vi "NIDAQControl.vi"() -> ()   [LabVIEW 2015]
uses:
  <vilib>/Analysis/NI_AALBase.lvlib
  NIDAQGlobals.vi
  <vilib>/Analysis/baseanly.llb/Mean (DBL).vi
  <vilib>/DAQmx/write.llb/DAQmx Write (Analog 1D Wfm NChan NSamp).vi
panel:
  in  "error out":errorcluster
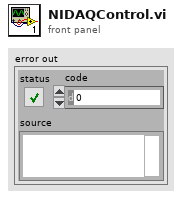
[diagram p1: front panel]
types:
  T1 = typedef "Rendezvous RefNum" = refnum<k1>
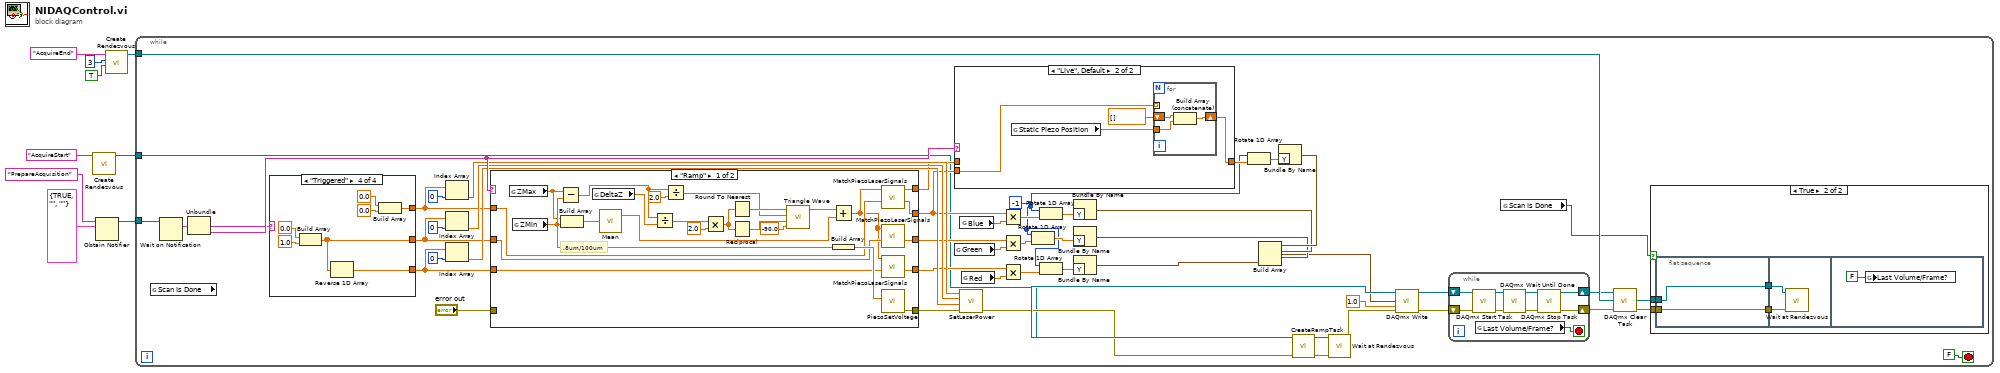
[diagram p0: block diagram]
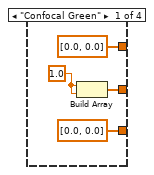
[diagram p4: hidden frame]
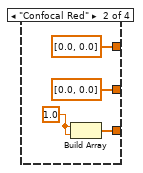
[diagram p5: hidden frame]
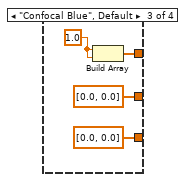
[diagram p6: hidden frame]
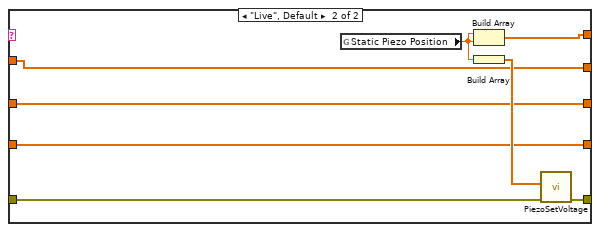
[diagram p7: hidden frame]
diagram:
  n1 = call <vilib>:"Create Rendezvous.vi"("name (unnamed)"="AcquireStart") -> ("rendezvous"=w5:T1)  [unwired: 4 in, 2 out]
  n2 = Obtain Notifier(name (unnamed)="PrepareAcquisition", notification data type=cluster{bool, string, string} {TRUE, "", ""}) -> (notifier out=w7:refnum<notifier>)  [unwired: 2 in, 2 out]
  n3 = call <vilib>:"Create Rendezvous.vi"("return existing (F)"=TRUE, "size (2)"=3, "name (unnamed)"="AcquireEnd") -> ("rendezvous"=w2:T1)  [unwired: 2 in, 2 out]
  n4 = while {
    tunnel: w7 -> [w58]
    tunnel: w5 -> [w37]
    tunnel: w2 -> [w36]
    stop <- FALSE stop-if-true
    w14 = -1 ("n")
    n5 = global read "NIDAQGlobals.vi" "Scan Is Done"() -> ()  [unwired: 1 out]
    n6 = Wait on Notification(notifier=w58) -> (notification=w57:cluster{bool, string, string})  [unwired: 3 in, 3 out]
    n7 = Unbundle(w57) -> (w54:string, w56:string)  [unwired: 1 out]
    n8 = case shown="\"Triggered\"" w54 {
      tunnel: [w88 dbl[] [0.0, 0.0] ("element") dbl[] [0.0, 0.0] ("element") w99] -> w43
      tunnel: [dbl[] [0.0, 0.0] ("element") dbl[] [0.0, 0.0] ("element") w95 w100] -> w44
      tunnel: [dbl[] [0.0, 0.0] ("element") w92 dbl[] [0.0, 0.0] ("element") w98] -> w42
      frame "Confocal Green" {
        w86 = 1.0 ("element")
        n9 = Build Array(w86, w86) -> (w88:dbl[])
      }
      frame "Confocal Red" {
        w90 = 1.0 ("element")
        n10 = Build Array(w90, w90) -> (w92:dbl[])
      }
      frame "Confocal Blue", Default {
        w94 = 1.0 ("element")
        n11 = Build Array(w94, w94) -> (w95:dbl[])
      }
      frame "Triggered" {
        n12 = Build Array(0.0 ("element"), 1.0 ("element")) -> (w99:dbl[])
        n13 = Reverse 1D Array(array=w99) -> (reversed array=w98:dbl[])
        n14 = Build Array(0.0 ("element"), 0.0 ("element")) -> (w100:dbl[])
      }
    }
    n15 = Index Array(array=w44, index=0) -> (element=w46:dbl)
    n16 = Index Array(array=w43, index=0) -> (element=w47:dbl)
    n17 = Index Array(array=w42, index=0) -> (element=w48:dbl)
    n18 = case shown="\"Ramp\"" w56 {
      tunnel: [w114 w136] -> w52
      tunnel: "error out" -> [_ w137]
      tunnel: [w107 w133] -> w38
      tunnel: w44 -> [w109 w131]
      tunnel: w43 -> [w110 w130]
      tunnel: w42 -> [w113 w132]
      tunnel: [w112 w132] -> w41
      tunnel: [w111 w130] -> w40
      tunnel: [w106 w131] -> w39
      frame "Ramp" {
        # ".8um/100um"
        n19 = global read "NIDAQGlobals.vi" "ZMax"() -> (w122:dbl)
        n20 = global read "NIDAQGlobals.vi" "ZMin"() -> (w123:dbl)
        n21 = Subtract(x=w122, y=w123) -> (x-y=w128:dbl)
        n22 = Build Array(w122, w123) -> (w125:dbl[])
        n23 = global read "NIDAQGlobals.vi" "DeltaZ"() -> (w121:dbl)
        n24 = call-poly <vilib>:"Mean.vi"("X"=w125) -> ("mean"=w116:dbl)  [unwired: 1 out]
        n25 = Divide(x=w128, y=w121) -> (x/y=w127:dbl)
        n26 = Divide(x=w128, y=2.0) -> (x/y=w115:dbl)
        n27 = Multiply(x=w127, y=2.0) -> (x*y=w105:dbl)
        n28 = Round To Nearest(number=w105) -> (nearest integer value=w118:dbl)
        n29 = Reciprocal(x=w105) -> (1/x=w117:dbl)
        n30 = call <vilib>:"Triangle Wave.vi"("samples"=w118, "amplitude"=w115, "frequency"=w117, "phase in"=-90.0) -> ("triangle wave"=w119:dbl[])  [unwired: 1 in, 2 out]
        n31 = Add(x=w119, y=w116) -> (x+y=w108:dbl[])
        n32 = Build Array(w123) -> (w124:dbl[])
        n33 = call "MatchPiezoLaserSignals.vi"("LaserSigIn"=w109, "PiezoSig"=w108) -> ("LaserSigOut"=w106:dbl[], "PiezoSigOut"=w107:dbl[])  [unwired: 7 in]
        n34 = call "MatchPiezoLaserSignals.vi"("LaserSigIn"=w110, "PiezoSig"=w108) -> ("LaserSigOut"=w111:dbl[])  [unwired: 7 in, 1 out]
        n35 = call "MatchPiezoLaserSignals.vi"("LaserSigIn"=w113, "PiezoSig"=w108) -> ("LaserSigOut"=w112:dbl[])  [unwired: 7 in, 1 out]
        n36 = call "PiezoSetVoltage.vi"("data"=w124) -> ("error out"=w114:errorcluster)  [unwired: 10 in]
      }
      frame "Live", Default {
        n37 = global read "NIDAQGlobals.vi" "Static Piezo Position"() -> (w134:dbl)
        n38 = Build Array(w134, w134) -> (w133:dbl[])
        n39 = Build Array(w134) -> (w135:dbl[])
        n40 = call "PiezoSetVoltage.vi"("error in"=w137, "data"=w135) -> ("error out"=w136:errorcluster)  [unwired: 9 in]
      }
    }
    n41 = case shown="\"Live\", Default" w56 {
      tunnel: w38 -> [w78 _]
      tunnel: w39 -> [_ w82]
      tunnel: [w78 w79] -> w28
      frame "Ramp" {
      }
      frame "Live", Default {
        n42 = global read "NIDAQGlobals.vi" "Static Piezo Position"() -> (w81:dbl)
        n43 = for {
          tunnel: w82 -> [_] mode=indexing
          tunnel: w81 -> [w83]
          shift-right: [w85] -> w79
          shift-left: dbl[] [] -> [w84]
          n44 = Build Array (concatenate)(w84, w83) -> (w85:dbl[])
        }
      }
    }
    n45 = global read "NIDAQGlobals.vi" "Green"() -> (w32:dbl)
    n46 = global read "NIDAQGlobals.vi" "Blue"() -> (w30:dbl)
    n47 = call "SetLaserPower.vi"("error in"=w52, "AOTF3"=w48, "AOTF2"=w47, "AOTF1"=w46) -> ("error out"=w45:errorcluster)  [unwired: 7 in]
    n48 = global read "NIDAQGlobals.vi" "Red"() -> (w34:dbl)
    n49 = Multiply(x=w39, y=w30) -> (x*y=w29:dbl[])
    n50 = Multiply(x=w40, y=w32) -> (x*y=w31:dbl[])
    n51 = Multiply(x=w41, y=w34) -> (x*y=w33:dbl[])
    n52 = Rotate 1D Array(1:w31, 2:w14) -> (0:w25:dbl[])
    n53 = Rotate 1D Array(1:w29, 2:w14) -> (0:w26:dbl[])
    n54 = Rotate 1D Array(1:w33, 2:w14) -> (0:w17:dbl[])
    n55 = Bundle By Name("Y"=w26) -> (w19:waveform(dbl))  [unwired: 1 in]
    n56 = Bundle By Name("Y"=w25) -> (w18:waveform(dbl))  [unwired: 1 in]
    n57 = Bundle By Name("Y"=w17) -> (w16:waveform(dbl))  [unwired: 1 in]
    n58 = Rotate 1D Array(1:w28, 2:w14) -> (0:w27:dbl[])
    n59 = Bundle By Name("Y"=w27) -> (w20:waveform(dbl))  [unwired: 1 in]
    n60 = Build Array(w20, w19, w18, w16) -> (w15:waveform(dbl)[])
    n61 = call "CreateRampTask.vi"("error in"=w45) -> ("error out"=w35:errorcluster, "task out"=w53:refnum<k21>)  [unwired: 9 in]
    n62 = call <vilib>:"Wait at Rendezvous.vi"("error in (no error)"=w35, "rendezvous"=w37) -> ("error out"=w24:errorcluster)  [unwired: 3 in, 2 out]
    n63 = call-poly <vilib>:"DAQmx Write.vi"("task/channels in"=w53, "data"=w15, "timeout"=1.0, "error in"=w24) -> ("task out"=w22:refnum<k21>, "error out"=w23:errorcluster)  [unwired: 9 in, 1 out]
    n64 = while {
      shift-right: [w70] -> w11
      shift-left: w23 -> [w73]
      shift-right: [w74] -> w13
      shift-left: w22 -> [w77]
      stop <- w69 stop-if-true
      n65 = call <vilib>:"DAQmx Start Task.vi"("task/channels in"=w77, "error in"=w73) -> ("task out"=w76:refnum<k21>, "error out"=w72:errorcluster)  [unwired: 12 in]
      n66 = global read "NIDAQGlobals.vi" "Last Volume/Frame?"() -> (w69:bool)
      n67 = call <vilib>:"DAQmx Wait Until Done.vi"("task/channels in"=w76, "error in"=w72) -> ("task out"=w75:refnum<k21>, "error out"=w71:errorcluster)  [unwired: 12 in]
      n68 = call <vilib>:"DAQmx Stop Task.vi"("task/channels in"=w75, "error in"=w71) -> ("task out"=w74:refnum<k21>, "error out"=w70:errorcluster)  [unwired: 12 in]
    }
    n69 = global read "NIDAQGlobals.vi" "Scan Is Done"() -> (w10:bool)
    n70 = call <vilib>:"DAQmx Clear Task.vi"("task in"=w13, "error in"=w11) -> ("error out"=w12:errorcluster)  [unwired: 13 in]
    n71 = case shown="True" w10 {
      tunnel: w36 -> [_ w61]
      tunnel: w12 -> [_ w60]
      frame False {
      }
      frame True {
        n72 = flat-sequence {
          tunnel: w61 -> [w65]
          tunnel: [w65] -> w63
          tunnel: [w64] -> w62
          tunnel: w60 -> [w64]
          tunnel: w63 -> [w67]
          tunnel: w62 -> [w66]
          frame #0 {
          }
          frame #1 {
            n73 = call <vilib>:"Wait at Rendezvous.vi"("error in (no error)"=w66, "rendezvous"=w67) -> ()  [unwired: 3 in, 3 out]
          }
          frame #2 {
            n74 = global write "NIDAQGlobals.vi" "Last Volume/Frame?"(FALSE ("Last Volume/Frame?")) -> ()
          }
        }
      }
    }
  }
